vi "Write Numeric Extensions.vi"(10 "Numeric Extensions (F)":bool, 11 "Serializer.JSON in":refnum<class "Serializer.JSON.lvclass">) -> (3 "Serializer.JSON out":refnum<class "Serializer.JSON.lvclass">)   [LabVIEW 2013, in "OpenSerializer.JKI-JSON.lvlib" / "Serializer.JSON.lvclass"]
uses:
  Serializer.JSON.lvclass
  Serializer.JSON.lvclass/Serializer.JSON.ctl
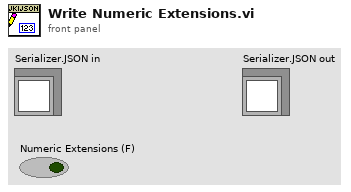
[diagram p1: front panel]
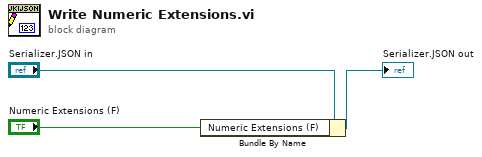
[diagram p0: block diagram]
diagram:
  n1 = Bundle By Name(cluster="Serializer.JSON in", "Numeric Extensions (F)"="Numeric Extensions (F)") -> (→"Serializer.JSON out":refnum<class "Serializer.JSON.lvclass">)
